vi "FES_CL_run.vi"() -> ()   [LabVIEW 2019]
uses:
  <vilib>/myRIO/Instrument Drivers/Onboard IO/DIO/typedefs/DIO Reference.ctl
  <vilib>/myRIO/Common/Instrument Driver Framework/Utilities/typedefs/myRIO Generic Hardware Reference.ctl
  <vilib>/myRIO/Common/Instrument Driver Framework/Utilities/typedefs/Hardware Version Enum.ctl
  <vilib>/myRIO/Common/Instrument Driver Framework/Utilities/typedefs/myRIO v1.0 Reference.ctl
  <vilib>/myRIO/Common/Instrument Driver Framework/Utilities/typedefs/Generic FPGA Reference.ctl
  <vilib>/myRIO/Common/Instrument Driver Framework/myRIO v1.0/DIO/typedefs/DIO Channels List.ctl
  <vilib>/myRIO/Common/Instrument Driver Framework/myRIO v1.0/DIO/typedefs/DIO Channels Enum.ctl
  <vilib>/userDefined/High Color/nirio_resource_hc.ctl
  <vilib>/Platform/TimedLoop/XDataNode/timing_clust.ctl
  <vilib>/Platform/TimedLoop/XDataNode/nitl_modes.ctl
  <vilib>/Platform/TimedLoop/XDataNode/wakeup.ctl
  <vilib>/myRIO/Instrument Drivers/Onboard IO/AI/typedefs/AI Reference.ctl
  <vilib>/myRIO/Common/Instrument Driver Framework/myRIO v1.0/AI/typedefs/AI Channels List.ctl
  <vilib>/myRIO/Common/Instrument Driver Framework/myRIO v1.0/AI/typedefs/AI Channels Enum.ctl
  <vilib>/myRIO/Common/Instrument Driver Framework/Utilities/typedefs/Analog Scaling Constants List.ctl
  <vilib>/myRIO/Common/Instrument Driver Framework/Utilities/typedefs/Analog Scaling Constants.ctl
  <vilib>/myRIO/Common/Instrument Driver Framework/Utilities/vis/Is FPGA Ref Available.vi
  <vilib>/myRIO/Common/Instrument Driver Framework/myRIO v1.0/DIO/vis/myRIO v1.1 Open DIO.vi
  <vilib>/myRIO/Instrument Drivers/Onboard IO/DIO/vis/Write.vi
  <vilib>/myRIO/Common/Instrument Driver Framework/myRIO v1.0/AI/vis/myRIO v1.1 Open AI.vi
  <vilib>/myRIO/Instrument Drivers/Onboard IO/AI/vis/Read.vi
  <vilib>/myRIO/Common/Instrument Driver Framework/Utilities/vis/Validate Channels.vi
  <vilib>/myRIO/Common/Instrument Driver Framework/myRIO v1.0/DIO/vis/myRIO v1.0 Reserve DIO.vi
  <vilib>/myRIO/Common/Instrument Driver Framework/myRIO v1.0/AI/vis/myRIO v1.0 Reserve AI.vi
  <vilib>/myRIO/Common/Instrument Driver Framework/myRIO v1.0/Resource Manager/vis/myRIO v1.0 Reserve Channel List.vi
  <vilib>/myRIO/Common/Instrument Driver Framework/myRIO v1.0/DIO/vis/myRIO v1.0 Build MUX Configuration DIO.vi
  <vilib>/myRIO/Common/Instrument Driver Framework/myRIO v1.0/AI/vis/myRIO v1.0 Build MUX Configuration AI.vi
  <vilib>/myRIO/Common/Instrument Driver Framework/myRIO v1.0/Resource Manager/vis/myRIO v1.0 Reserve Channel.vi
  <vilib>/myRIO/Common/Instrument Driver Framework/myRIO v1.0/Resource Manager/vis/myRIO v1.0 Unreserve Channel.vi
  <vilib>/myRIO/Common/Instrument Driver Framework/myRIO v1.0/Resource Manager/vis/myRIO v1.0 Create Configuration List.vi
  <vilib>/myRIO/Common/Instrument Driver Framework/myRIO v1.0/Resource Manager/vis/myRIO v1.0 Build Mutex Name.vi
  <vilib>/Utility/VariantDataType/GetNumericInfo.vi
  <vilib>/Utility/error.llb/Error Cluster From Error Code.vi
  <vilib>/myRIO/Common/Instrument Driver Framework/myRIO v1.0/myRIO v1.1 Open.vi
  <vilib>/myRIO/Common/Instrument Driver Framework/Utilities/vis/IO Manager.vi
  <vilib>/myRIO/Common/Instrument Driver Framework/Utilities/vis/Configuration Manager.vi
  <vilib>/myRIO/Common/Instrument Driver Framework/myRIO v1.0/Resource Manager/vis/myRIO v1.0 Configure IO.vi
  <vilib>/myRIO/Common/Instrument Driver Framework/myRIO v1.0/myRIO v1.0 Close.vi
  <vilib>/myRIO/Common/Instrument Driver Framework/myRIO v1.0/DIO/vis/myRIO v1.0 Write DIO.vi
  <vilib>/Utility/file.llb/Read Delimited Spreadsheet (DBL).vi
  FOS_CL/Global_vars.vi
  <vilib>/Utility/file.llb/Write Delimited Spreadsheet (DBL).vi
  <vilib>/myRIO/Common/Instrument Driver Framework/myRIO v1.0/AI/vis/myRIO v1.0 Get Scaling Constants AI.vi
  <vilib>/myRIO/Common/Instrument Driver Framework/myRIO v1.0/AI/vis/myRIO v1.0 Read AI.vi
  <vilib>/addons/control/pid/pid.llb/PID (DBL).vi
  <vilib>/myRIO/Express VI/Onboard IO/DO/DO Express VI.xnode
  <vilib>/myRIO/Instrument Drivers/Onboard IO/DIO/vis/myRIO DIO Open.xnode
  <vilib>/Platform/TimedLoop/XDataNode/XDataNode.xnode
  <vilib>/myRIO/Express VI/Onboard IO/AI/AI Express VI.xnode
  <vilib>/myRIO/Instrument Drivers/Onboard IO/AI/vis/myRIO AI Open.xnode
  <vilib>/myRIO/Instrument Drivers/Onboard IO/DIO/DIO.lvlib
  <vilib>/Platform/TimedLoop/XDataNode/XDNodeRunTimeDep.lvlib
  <vilib>/myRIO/Instrument Drivers/Onboard IO/AI/AI.lvlib
  <vilib>/ptbypt/NI_PtbyPt.lvlib
  <vilib>/addons/control/pid/NI_PID_pid.lvlib
panel:
  in  "Setup":T1(tab)
  in  "Sin Sq":bool
  in  "Ref freq (Hz)":dbl
  in  "Ref amp (mN)":dbl
  in  "Offset (mN)":dbl
  in  "output range":cluster{"output high":dbl, "output low":dbl}={"output high"=100.0, "output low"=-100.0} {"output low" format="%.2f"; "output high" format="%.2f"}
  in  "PID gains":T2={"proportional gain (Kc)"=1.0, "integral time (Ti, min)"=0.01, "derivative time (Td, min)"=0.0} {"derivative time (Td, min)" format="%.3f"; "integral time (Ti, min)" format="%.3f"; "proportional gain (Kc)" format="%.3f"}
  in  "Gyk":dbl
  in  "maxCS":dbl
  in  "minCS":dbl
  in  "Gff":dbl
  in  "y2":dbl
  in  "y1":dbl
  in  "x0":dbl
  in  "x1":dbl
  in  "x2":dbl
  in  "Offset2 (mN)":dbl
  in  "delta force (mN)":dbl
  in  "PW test (0-100%)":dbl
  in  "Stim Frequency (Hz)":dbl=39.0
  out "feedforward missed":dbl
  out "controller missed":dbl
  out "stim missed":dbl
  out "force reading missed":dbl
  out "save missed":dbl
  out "ref missed":dbl
  out "Fref":dbl[](graph)
  in  "File path":path=path "C:/Opto/fatigue_plantar2.txt"
  out "Control performance":cluster{"F ref":dbl, "raw F":dbl}(graph)
  out "Control signal":dbl(graph)
  out "forceInd":dbl
  out "Control signals":T3(graph)
  out "yk":dbl(graph)
  in  "Mode test CL":bool
  in  "stop":bool
  in  "Model off on":bool
  out "rawF":dbl[](graph)
  in  "stop test":bool
  out "controlSignal":dbl[](graph)
  out "controlVariable":dbl[](graph)
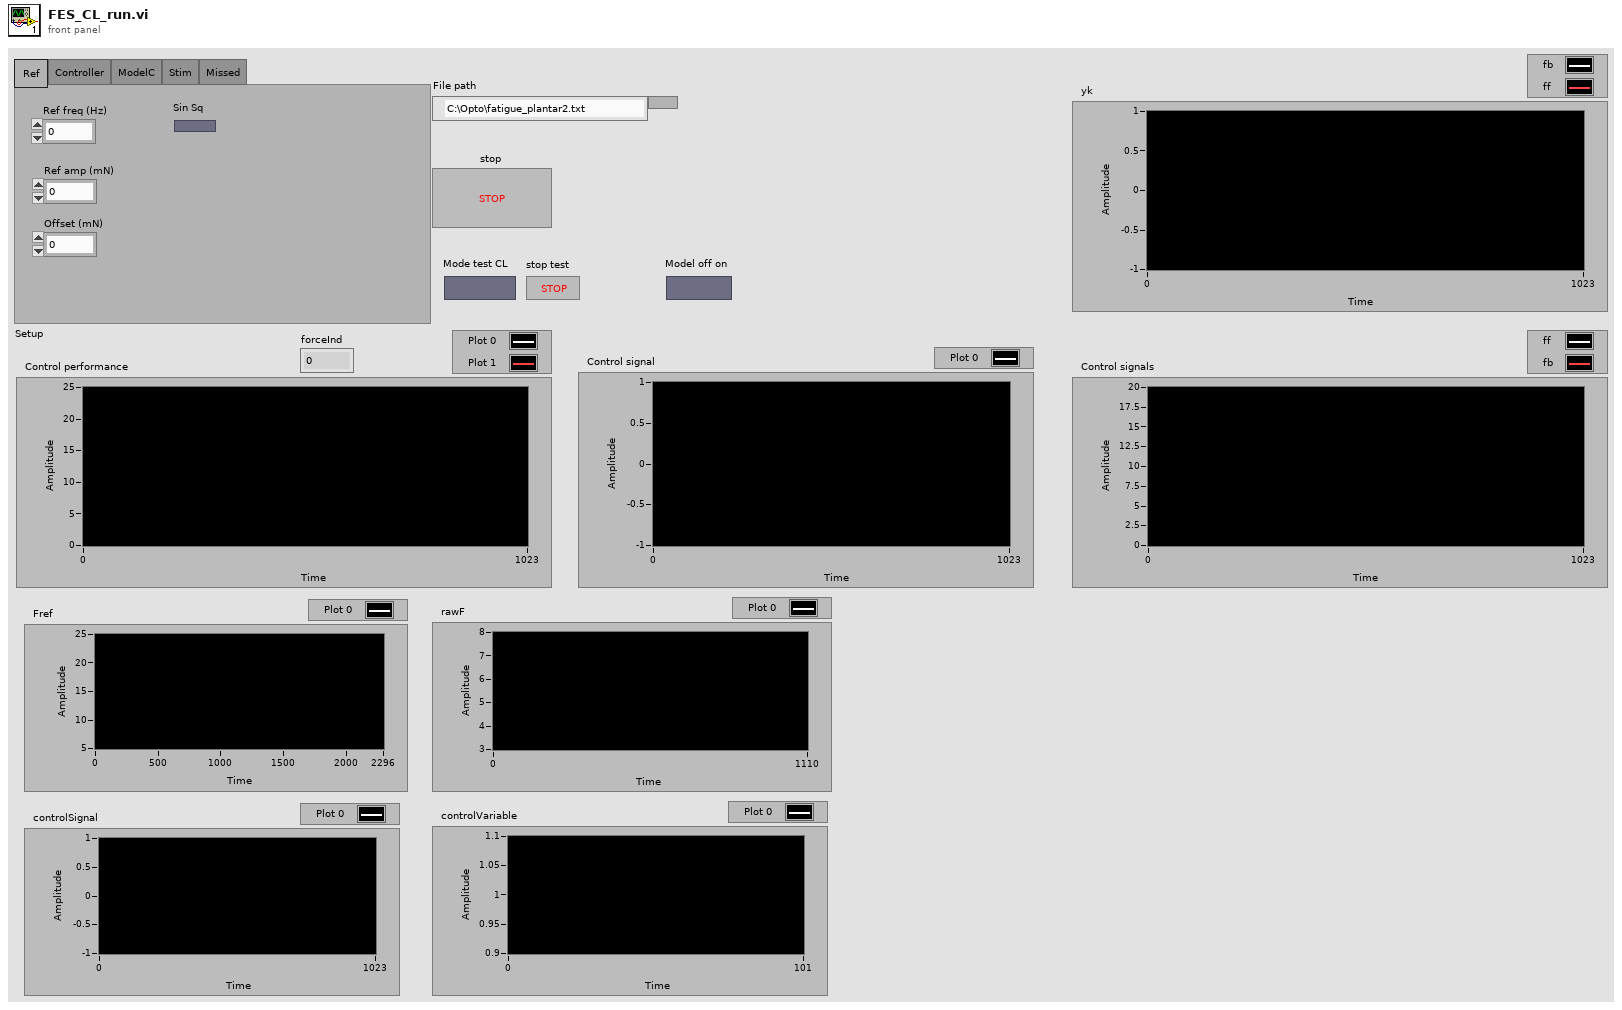
[diagram p1: front panel]
types:
  T1 = enum32{"Ref ", "Controller", "ModelC", "Stim", "Missed"}
  T2 = cluster{"proportional gain (Kc)":dbl, "integral time (Ti, min)":dbl, "derivative time (Td, min)":dbl}
  T3 = cluster{"control signal ff":dbl, "control signal fb":dbl}
  T4 = typedef "DIO.lvlib/DIO Reference.ctl" = cluster{"myRIO Reference":T5, "DIO Channels List":T9}
  T5 = typedef "myRIO Generic Hardware Reference.ctl" = cluster{"myRIO Model":T6, "myRIO Hardware Reference":T7}
  T6 = typedef "Hardware Version Enum.ctl" = enum16{"Unknown", "myRIO-1900", "myRIO-1950", "roboRIO", "NI ELVIS RIO CM", "ELVIS III"}
  T7 = typedef "myRIO v1.0 Reference.ctl" = cluster{"Generic FPGA Reference":T8, "Allow multiple opens":bool}
  T8 = typedef "Generic FPGA Reference.ctl" = refnum<k20>
  T9 = typedef "DIO Channels List.ctl" = T10[]
  T10 = typedef "DIO Channels Enum.ctl" = enum16{"Not Connected", "C/DIO0", "C/DIO1", "C/DIO2", "C/DIO3", "C/DIO4", "C/DIO5", "C/DIO6", "C/DIO7", "A/DIO0", "A/DIO1", "A/DIO2", "A/DIO3", "A/DIO4", "A/DIO5", "A/DIO6", "A/DIO7", "A/DIO8", "A/DIO9", "A/DIO10", "A/DIO11", "A/DIO12", "A/DIO13", "A/DIO14", "A/DIO15", "A/DIO16", "A/DIO17", "A/DIO18", "A/DIO19", "B/DIO0", "B/DIO1", "B/DIO2", "B/DIO3", "B/DIO4", "B/DIO5", "B/DIO6", "B/DIO7", "B/DIO8", "B/DIO9", "B/DIO10", "B/DIO11", "B/DIO12", "B/DIO13", "B/DIO14", "B/DIO15", "B/DIO16", "B/DIO17", "B/DIO18", "B/DIO19", "LED0", "LED1", "LED2", "LED3", "Button0", "DIO/DIO0", "DIO/DIO1", "DIO/DIO2", "DIO/DIO3", "DIO/DIO4", "DIO/DIO5", "DIO/DIO6", "DIO/DIO7", "DIO/DIO8", "DIO/DIO9", "SPI/CS0", "SPI/CS1", "SPI/CS2", "SPI/CS3", "LED RADIO (Green)", "LED RADIO (Red)", "LED COMM (Green)", "LED COMM (Red)", "LED MODE (Green)", "LED MODE (Red)"}
  T11 = typedef "nirio_resource_hc.ctl" = tag
  T12 = typedef "XDNodeRunTimeDep.lvlib/timing_clust.ctl" = cluster{"Expected End [f-1]":u64, "Actual End [f-1]":u64, "Finished Late? [f-1]":bool, "Expected End [i-1]":u64, "Actual End [i-1]":u64, "Finished Late? [i-1]":bool, "Expected Start [i]":u64, "Actual Start [i]":u64, "Expected Start [f]":u64, "Actual Start [f]":u64, "Source Name":string, "Structure Name":string, "Period":i64, "Deadline":i64, "Offset":i64, "Start":i64, "Priority":i32, "Timeout":i32, "Mode":T13, "Wakeup Reason":T14, "Error":errorcluster, "Source Type":string, "Secondary Source Type":string, "Global End Time":u64, "Global Start Time":u64, "Frame Duration":u64, "Iteration Duration":u64, "Assigned CPU":i32, "I/O Scan Engine Mode":u32}
  T13 = typedef "XDNodeRunTimeDep.lvlib/nitl_modes.ctl" = enum32{"No Change", "Process missed periods, maintain original phase", "Discard missed periods, maintain original phase", "Process missed periods, ignore original phase", "Discard missed periods, ignore original phase"}
  T14 = typedef "XDNodeRunTimeDep.lvlib/wakeup.ctl" = enum32{"Normal", "Aborted", "Asynchronous wakeup", "Timing source error", "Timed loop error", "Timeout"}
  T15 = typedef "AI.lvlib/AI Reference.ctl" = cluster{"myRIO Reference":T5, "AI Channels List":T16, "AI Scaling Constants List":T18}
  T16 = typedef "AI Channels List.ctl" = T17[]
  T17 = typedef "AI Channels Enum.ctl" = enum16{"Not Connected", "AudioIn/Left", "AudioIn/Right", "C/AI0", "C/AI1", "A/AI0", "A/AI1", "A/AI2", "A/AI3", "A/AI4", "A/AI5", "A/AI6", "A/AI7", "B/AI0", "B/AI1", "B/AI2", "B/AI3", "B/AI4", "B/AI5", "B/AI6", "B/AI7", "AI/AI0", "AI/AI1", "AI/AI2", "AI/AI3", "A/AI0 (DIFF)", "A/AI1 (DIFF)", "A/AI2 (DIFF)", "A/AI3 (DIFF)", "B/AI0 (DIFF)", "B/AI1 (DIFF)", "B/AI2 (DIFF)", "B/AI3 (DIFF)"}
  T18 = typedef "Analog Scaling Constants List.ctl" = T19[]
  T19 = typedef "Analog Scaling Constants.ctl" = cluster{"LSB Weight (Volts)":dbl, "Offset (Volts)":dbl, "Signed?":bool}
  T20 = cluster{"control signal fb":dbl, "control signal ff":dbl}
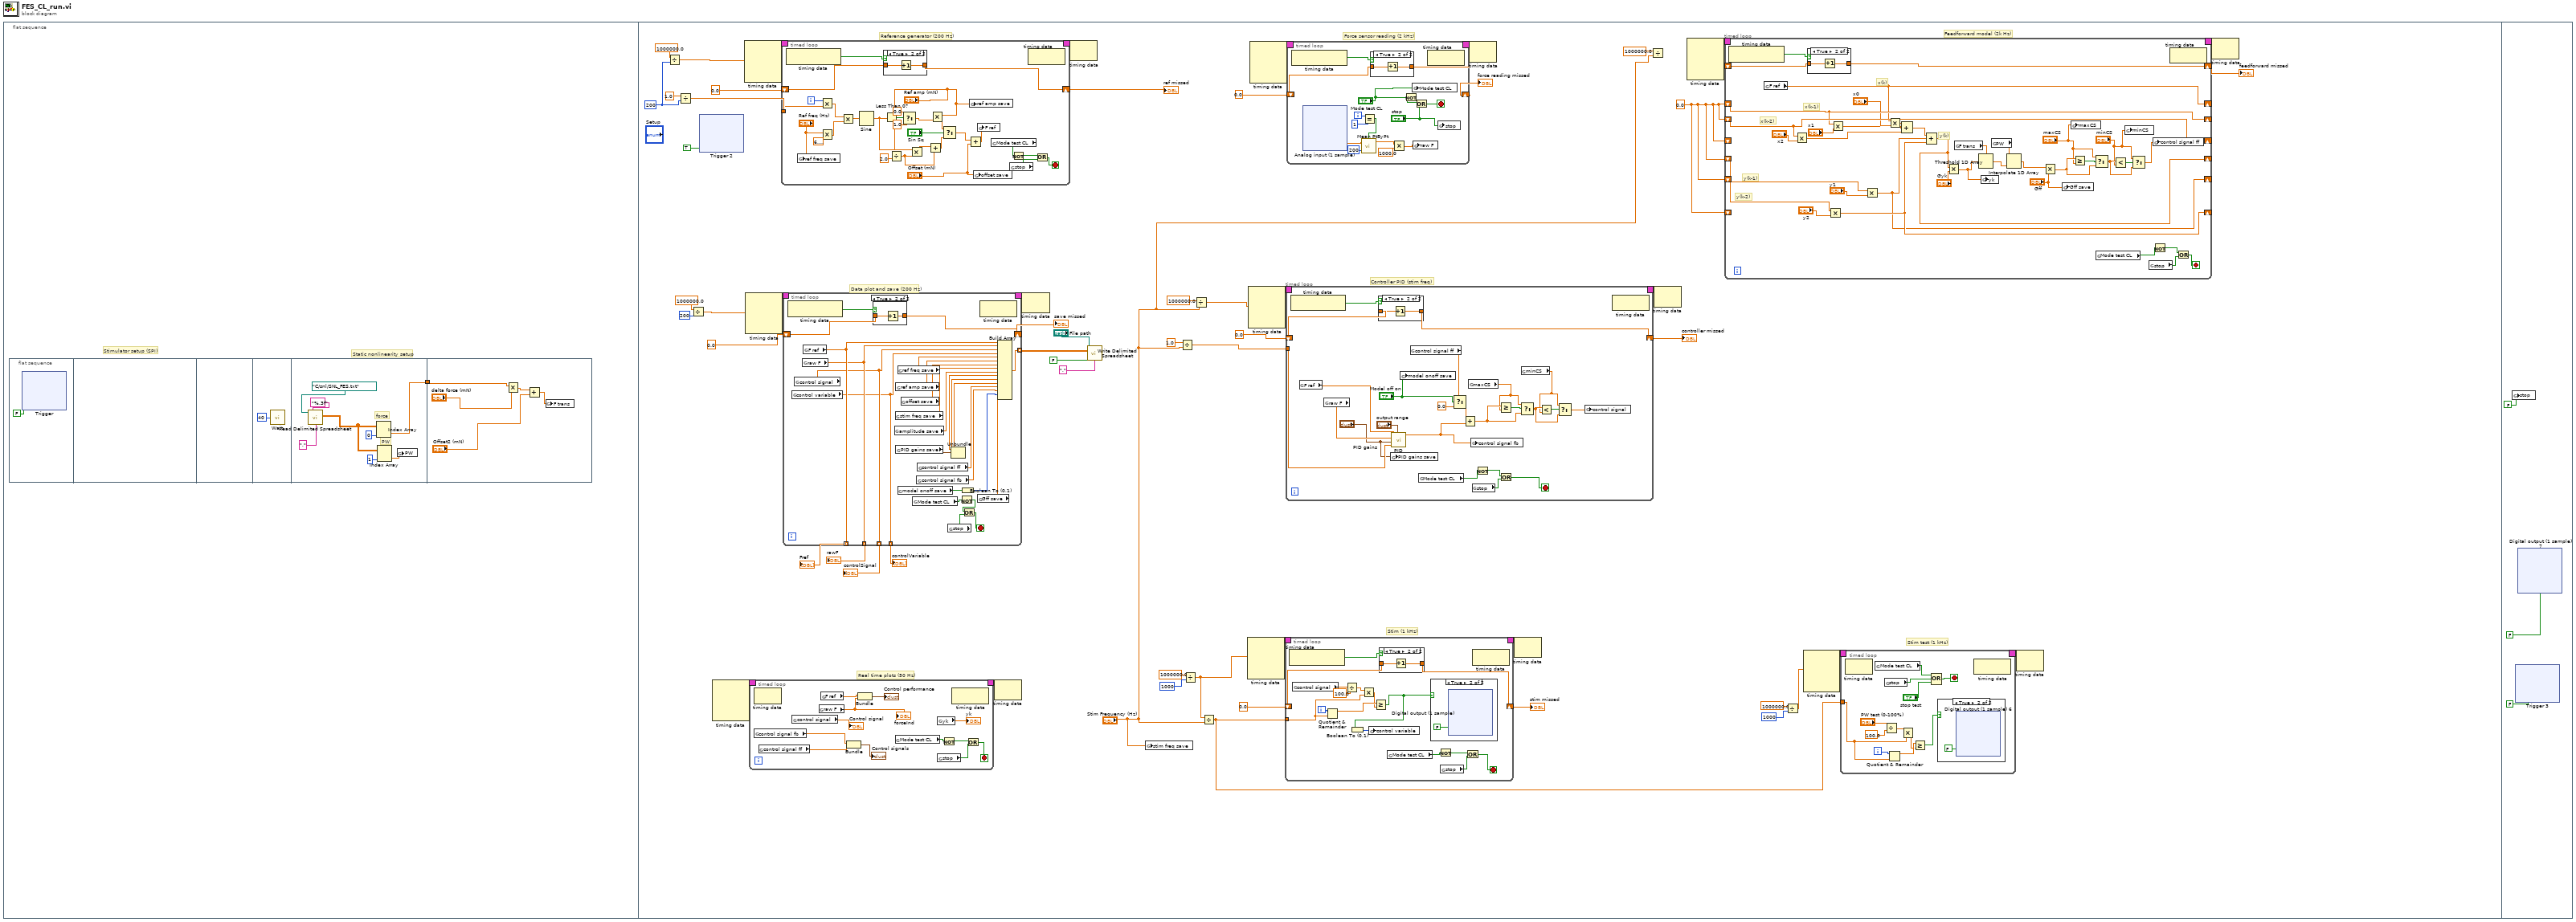
[diagram p0: block diagram]
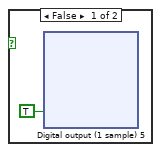
[diagram p3: hidden frame]
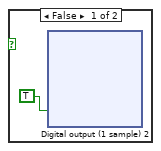
[diagram p5: hidden frame]
diagram:
  n1 = flat-sequence {
    frame #0 {
      # "Static nonlinearity setup"
      # "Stimulator setup (SPI)"
      n2 = flat-sequence {
        tunnel: [w39] -> w1
        tunnel: w1 -> [w50]
        frame #0 {
          n3 = xnode "Trigger"("C/DIO7 (DIO7)"=FALSE) -> ()  [unwired: 1 in, 1 out]
        }
        frame #1 {
        }
        frame #2 {
        }
        frame #3 {
          n4 = call "Wait"("Count(uSec)"=u32 40) -> ()  [unwired: 1 out]
        }
        frame #4 {
          # "PW"
          # "force"
          n5 = call-poly <vilib>:"Read Delimited Spreadsheet.vi"("file path (dialog if empty)"=path "C:/snl/SNL_FES.txt", "format (%.3f)"="%.3f", "delimiter (\\t)"="," ("delimiter (\\t)")) -> ("all rows"=w45:dbl[][])  [unwired: 7 in, 5 out]
          n6 = Index Array(array=w45, index (col)=0 ("disabled index (col)")) -> (element=w39:dbl[])  [unwired: 1 in]
          n7 = Index Array(array=w45, index (col)=1 ("disabled index (col)")) -> (element=w46:dbl[])  [unwired: 1 in]
          n8 = global write "Global_vars.vi" "PW"(w46) -> ()
        }
        frame #5 {
          n9 = Multiply(x=w50, y="delta force (mN)") -> (x*y=w51:dbl[])
          n10 = Add(x=w51, y="Offset2 (mN)") -> (x+y=w49:dbl[])
          n11 = global write "Global_vars.vi" "F trans"(w49) -> ()
        }
      }
    }
    frame #1 {
      w56 = 0.0 ("F ref")
      w101 = 200
      # "Feedforward model (2k Hz)"
      # "Stim test (1 kHz)"
      # "Stim (1 kHz)"
      # "Controller PID (stim freq)"
      # "Force sensor reading (2 kHz)"
      # "Real time plots (50 Hz)"
      # "Data plot and save (200 Hz)"
      # "Reference generator (200 Hz)"
      n12 = Divide(x=1000000.0, y=w101) -> (x/y=w103:dbl)
      n13 = Divide(x=1.0, y=w101) -> (x/y=w106:dbl)
      n14 = Divide(x=1000000.0, y=200) -> (x/y=w100:dbl)
      n15 = xnode "Trigger 2"("C/DIO7 (DIO7)"=TRUE) -> ()  [unwired: 1 in, 1 out]
      n16 = node-c288() -> (w93:T12)  [unwired: 4 in]
      n17 = node-c288(w103) -> (w109:T12)  [unwired: 3 in]
      n18 = node-c288(w100) -> (w105:T12)  [unwired: 3 in]
      n19 = timed-loop {
        timing: w93 -> [_]
        timing-out: [_] -> w92
        stop <- w481 stop-if-true
        n20 = node-c288() -> ()  [unwired: 1 in, 1 out]
        n21 = global read "Global_vars.vi" "control signal fb"() -> (w475:dbl)
        n22 = global read "Global_vars.vi" "control signal ff"() -> (w474:dbl)
        n23 = global read "Global_vars.vi" "control signal"() -> (→"Control signal":dbl)
        n24 = global read "Global_vars.vi" "raw F"() -> (w477:dbl)
        "forceInd" <- w477
        n25 = global read "Global_vars.vi" "F ref"() -> (w478:dbl)
        n26 = Bundle("control signal fb"=w475, "control signal ff"=w474) -> (→"Control signals":T20)  [unwired: 1 in]
        n27 = Bundle("F ref"=w478, "raw F"=w477) -> (→"Control performance":cluster{"F ref":dbl, "raw F":dbl})  [unwired: 1 in]
        n28 = global read "Global_vars.vi" "Mode test CL"() -> (w484:bool)
        n29 = global read "Global_vars.vi" "yk"() -> (→"yk":dbl)
        n30 = global read "Global_vars.vi" "stop"() -> (w482:bool)
        n31 = Not(x=w484) -> (.not. x?=w483:bool)
        n32 = node-c288() -> ()  [unwired: 1 in, 1 out]
        n33 = Or(x=w483, y=w482) -> (x .or. y?=w481:bool)
      }
      n34 = timed-loop {
        timing: w109 -> [_]
        timing-out: [_] -> w108
        tunnel: w106 -> [w551]
        shift-right: [w532] -> w90
        shift-left: 0.0 -> [w533]
        i -> [w552]
        stop <- w531 stop-if-true
        n35 = node-c288() -> (w534:bool)  [unwired: 1 in]
        n36 = global write "Global_vars.vi" "ref freq save"("Ref freq (Hz)") -> ()
        n37 = Multiply(x=w552, y=w551) -> (x*y=w550:dbl)
        n38 = Multiply(x="Ref freq (Hz)", y=6.283185307179586) -> (x*y=w549:dbl)
        n39 = Multiply(x=w550, y=w549) -> (x*y=w548:dbl)
        n40 = Sine(x=w548) -> (sin(x)=w539:dbl)
        n41 = case shown="True" w534 {
          tunnel: w533 -> [w554 w556]
          tunnel: [w554 w555] -> w532
          frame False {
          }
          frame True {
            n42 = Increment(x=w556) -> (x+1=w555:dbl)
          }
        }
        n43 = Less Than 0?(x=w539) -> (x < 0?=w547:bool)
        n44 = Divide(x="Ref amp (mN)", y=2.0) -> (x/y=w538:dbl)
        n45 = Select(t=0.0, s=w547, f=1.0) -> (s? t:f=w542:dbl)
        n46 = Multiply(x=w539, y=w538) -> (x*y=w537:dbl)
        n47 = Add(x=w537, y=w538) -> (x+y=w536:dbl)
        n48 = Multiply(x="Ref amp (mN)", y=w542) -> (x*y=w541:dbl)
        n49 = Select(t=w541, s="Sin Sq", f=w536) -> (s? t:f=w535:dbl)
        n50 = Add(x=w535, y="Offset (mN)") -> (x+y=w543:dbl)
        n51 = global write "Global_vars.vi" "ref amp save"("Ref amp (mN)") -> ()
        n52 = global write "Global_vars.vi" "offset save"("Offset (mN)") -> ()
        n53 = global write "Global_vars.vi" "F ref"(w543) -> ()
        n54 = global read "Global_vars.vi" "Mode test CL"() -> (w529:bool)
        n55 = global read "Global_vars.vi" "stop"() -> (w530:bool)
        n56 = Not(x=w529) -> (.not. x?=w528:bool)
        n57 = node-c288() -> ()  [unwired: 1 in, 1 out]
        n58 = Or(x=w528, y=w530) -> (x .or. y?=w531:bool)
      }
      "ref missed" <- w90
      n59 = timed-loop {
        timing: w105 -> [_]
        timing-out: [_] -> w104
        tunnel: [w511] -> w96 mode=indexing
        shift-right: [w512] -> w88
        shift-left: 0.0 -> [w513]
        tunnel: [w510] -> w69 mode=indexing
        tunnel: [w509] -> w68 mode=indexing
        tunnel: [w504] -> w61 mode=indexing
        tunnel: [w503] -> w60 mode=indexing
        stop <- w507 stop-if-true
        n60 = node-c288() -> (w514:bool)  [unwired: 1 in]
        n61 = global read "Global_vars.vi" "control variable"() -> (w503:dbl)
        n62 = global read "Global_vars.vi" "control signal"() -> (w504:dbl)
        n63 = global read "Global_vars.vi" "raw F"() -> (w510:dbl)
        n64 = global read "Global_vars.vi" "F ref"() -> (w511:dbl)
        n65 = case shown="True" w514 {
          tunnel: w513 -> [w515 w517]
          tunnel: [w515 w516] -> w512
          frame False {
          }
          frame True {
            n66 = Increment(x=w517) -> (x+1=w516:dbl)
          }
        }
        n67 = global read "Global_vars.vi" "amplitude save"() -> (w498:dbl)
        n68 = global read "Global_vars.vi" "stim freq save"() -> (w499:dbl)
        n69 = global read "Global_vars.vi" "ref amp save"() -> (w501:dbl)
        n70 = global read "Global_vars.vi" "PID gains save"() -> (w497:T2)
        n71 = global read "Global_vars.vi" "ref freq save"() -> (w502:dbl)
        n72 = global read "Global_vars.vi" "model onoff save"() -> (w491:bool)
        n73 = global read "Global_vars.vi" "offset save"() -> (w500:dbl)
        n74 = global read "Global_vars.vi" "Mode test CL"() -> (w505:bool)
        n75 = global read "Global_vars.vi" "control signal fb"() -> (w492:dbl)
        n76 = global read "Global_vars.vi" "control signal ff"() -> (w493:dbl)
        n77 = global read "Global_vars.vi" "stop"() -> (w508:bool)
        n78 = Unbundle(w497) -> ("proportional gain (Kc)"=w496:dbl, "integral time (Ti, min)"=w495:dbl, "derivative time (Td, min)"=w494:dbl)
        n79 = Not(x=w505) -> (.not. x?=w506:bool)
        n80 = Boolean To (0,1)(Boolean=w491) -> (0, 1=w490:i16)
        n81 = Or(x=w506, y=w508) -> (x .or. y?=w507:bool)
        n82 = global read "Global_vars.vi" "Gff save"() -> (w489:dbl)
        n83 = node-c288() -> ()  [unwired: 1 in, 1 out]
        n84 = Build Array(w511, w510, w504, w503, w502, w501, w500, w499, w498, w496, w495, w494, w493, w492, w490, w489) -> (w509:dbl[])
      }
      "Fref" <- w96
      "save missed" <- w88
      "rawF" <- w69
      "controlSignal" <- w61
      "controlVariable" <- w60
      n85 = node-c288(w92) -> ()  [unwired: 1 out]
      n86 = node-c288(w104) -> ()  [unwired: 1 out]
      n87 = node-c288(w108) -> ()  [unwired: 1 out]
      n88 = call-poly <vilib>:"Write Delimited Spreadsheet.vi"("file path (dialog if empty)"="File path", "2D data"=w68, "append to file? (new file:F)"=FALSE, "delimiter (\\t)"="," ("delimiter (\\t)")) -> ()  [unwired: 10 in, 2 out]
      n89 = global write "Global_vars.vi" "stim freq save"("Stim Frequency (Hz)") -> ()
      n90 = Divide(x=1.0, y="Stim Frequency (Hz)") -> (x/y=w72:dbl)
      n91 = Divide(x=1000000.0, y=1000) -> (x/y=w77:dbl)
      n92 = Divide(x=1000000.0, y="Stim Frequency (Hz)") -> (x/y=w52:dbl)
      n93 = Divide(x=w77, y="Stim Frequency (Hz)") -> (x/y=w62:dbl)
      n94 = node-c288(w77) -> (w81:T12)  [unwired: 3 in]
      n95 = node-c288(w52) -> (w83:T12)  [unwired: 3 in]
      n96 = node-c288() -> (w87:T12)  [unwired: 4 in]
      n97 = timed-loop {
        timing: w81 -> [_]
        timing-out: [_] -> w80
        tunnel: w62 -> [w293]
        shift-right: [w290] -> w75
        shift-left: 0.0 -> [w291]
        i -> [w292]
        stop <- w284 stop-if-true
        n98 = node-c288() -> (w289:bool)  [unwired: 1 in]
        n99 = global read "Global_vars.vi" "control signal"() -> (w296:dbl)
        n100 = Quotient & Remainder(x=w292, y=w293) -> (x-y*floor(x/y)=w282:dbl)  [unwired: 1 out]
        n101 = Divide(x=w296, y=100.0) -> (x/y=w294:dbl)
        n102 = Multiply(x=w294, y=w293) -> (x*y=w281:dbl)
        n103 = Greater Or Equal?(x=w282, y=w281) -> (x >= y?=w288:bool)
        n104 = Boolean To (0,1)(Boolean=w288) -> (0, 1=w287:i16)
        n105 = global write "Global_vars.vi" "control variable"(w287) -> ()
        n106 = case shown="True" w289 {
          tunnel: w291 -> [w297 w299]
          tunnel: [w297 w298] -> w290
          frame False {
          }
          frame True {
            n107 = Increment(x=w299) -> (x+1=w298:dbl)
          }
        }
        n108 = global read "Global_vars.vi" "Mode test CL"() -> (w283:bool)
        n109 = case shown="True" w288 {
          frame False {
            n110 = xnode "Digital output (1 sample) 2"("CH1 (C/DIO7 (DIO7))"=TRUE ("CH1 (A/DIO8 (Pin 27))")) -> ()  [unwired: 1 in, 1 out]
          }
          frame True {
            n111 = xnode "Digital output (1 sample)"("CH1 (C/DIO7 (DIO7))"=FALSE ("CH1 (A/DIO8 (Pin 27))")) -> ()  [unwired: 1 in, 1 out]
          }
        }
        n112 = Not(x=w283) -> (.not. x?=w285:bool)
        n113 = global read "Global_vars.vi" "stop"() -> (w286:bool)
        n114 = Or(x=w285, y=w286) -> (x .or. y?=w284:bool)
        n115 = node-c288() -> ()  [unwired: 1 in, 1 out]
      }
      "stim missed" <- w75
      n116 = timed-loop {
        timing: w83 -> [_]
        timing-out: [_] -> w82
        tunnel: w72 -> [w400]
        shift-right: [w397] -> w70
        shift-left: 0.0 -> [w398]
        stop <- w394 stop-if-true
        n117 = node-c288() -> (w399:bool)  [unwired: 1 in]
        n118 = global read "Global_vars.vi" "F ref"() -> (w389:dbl)
        n119 = global read "Global_vars.vi" "raw F"() -> (w401:dbl)
        n120 = case shown="True" w399 {
          tunnel: w398 -> [w403 w405]
          tunnel: [w403 w404] -> w397
          frame False {
          }
          frame True {
            n121 = Increment(x=w405) -> (x+1=w404:dbl)
          }
        }
        n122 = global write "Global_vars.vi" "PID gains save"("PID gains") -> ()
        n123 = call-poly <vilib>:"PID.vi"("output range"="output range", "dt (s)"=w400, "PID gains"="PID gains", "process variable"=w401, "setpoint"=w389) -> ("output"=w379:dbl)  [unwired: 5 in, 1 out]
        n124 = global write "Global_vars.vi" "model onoff save"("Model off on") -> ()
        n125 = global read "Global_vars.vi" "control signal ff"() -> (w388:dbl)
        n126 = global read "Global_vars.vi" "Mode test CL"() -> (w393:bool)
        n127 = Select(t=w388, s="Model off on", f=0.0) -> (s? t:f=w390:dbl)
        n128 = Add(x=w390, y=w379) -> (x+y=w382:dbl)
        n129 = global read "Global_vars.vi" "maxCS"() -> (w381:dbl)
        n130 = global write "Global_vars.vi" "control signal fb"(w379) -> ()
        n131 = global read "Global_vars.vi" "stop"() -> (w396:bool)
        n132 = Not(x=w393) -> (.not. x?=w395:bool)
        n133 = Greater Or Equal?(x=w382, y=w381) -> (x >= y?=w386:bool)
        n134 = Or(x=w395, y=w396) -> (x .or. y?=w394:bool)
        n135 = Select(t=w381, s=w386, f=w382) -> (s? t:f=w384:dbl)
        n136 = global read "Global_vars.vi" "minCS"() -> (w380:dbl)
        n137 = Less?(x=w384, y=w380) -> (x < y?=w385:bool)
        n138 = Select(t=w380, s=w385, f=w384) -> (s? t:f=w383:dbl)
        n139 = global write "Global_vars.vi" "control signal"(w383) -> ()
        n140 = node-c288() -> ()  [unwired: 1 in, 1 out]
      }
      "controller missed" <- w70
      n141 = timed-loop {
        timing: w87 -> [_]
        timing-out: [_] -> w86
        shift-right: [w421] -> w84
        shift-left: 0.0 -> [w422]
        i -> [w426]
        stop <- w418 stop-if-true
        n142 = node-c288() -> (w423:bool)  [unwired: 1 in]
        n143 = xnode "Analog input (1 sample)"() -> ("C/AI0 (AI0)"=w413:dbl)  [unwired: 1 in, 1 out]
        n144 = Equal?(x=w426, y=1) -> (x = y?=w424:bool)
        n145 = call <vilib>:"Mean PtByPt.vi"("x"=w413, "sample length"=200, "initialize"=w424) -> ("mean"=w415:dbl)  [unwired: 1 in, 1 out]
        n146 = case shown="True" w423 {
          tunnel: w422 -> [w428 w430]
          tunnel: [w428 w429] -> w421
          frame False {
          }
          frame True {
            n147 = Increment(x=w430) -> (x+1=w429:dbl)
          }
        }
        n148 = Multiply(x=w415, y=1000.0) -> (x*y=w414:dbl)
        n149 = Not(x="Mode test CL") -> (.not. x?=w420:bool)
        n150 = global write "Global_vars.vi" "Mode test CL"("Mode test CL") -> ()
        n151 = global write "Global_vars.vi" "raw F"(w414) -> ()
        n152 = Or(x=w420, y="stop") -> (x .or. y?=w418:bool)
        n153 = node-c288() -> ()  [unwired: 1 in, 1 out]
        n154 = global write "Global_vars.vi" "stop"("stop") -> ()
      }
      "force reading missed" <- w84
      n155 = node-c288(w86) -> ()  [unwired: 1 out]
      n156 = node-c288(w80) -> ()  [unwired: 1 out]
      n157 = Divide(x=1000000.0, y="Stim Frequency (Hz)") -> ()  [unwired: 1 out]
      n158 = node-c288(w82) -> ()  [unwired: 1 out]
      n159 = node-c288() -> (w58:T12)  [unwired: 4 in]
      n160 = timed-loop {
        timing: w58 -> [_]
        timing-out: [_] -> w57
        shift-right: [w145] -> w55
        shift-left: _ -> [w146]
        shift-right: [w111] -> _
        shift-left: w56 -> [w124]
        shift-right: [w124] -> _
        shift-left: w56 -> [w126]
        shift-right: [w126] -> _
        shift-left: w56 -> [_]
        shift-right: [w112] -> _
        shift-left: w56 -> [w134]
        shift-right: [w135] -> _
        shift-left: w56 -> [w139]
        shift-right: [w136] -> _
        shift-left: w56 -> [_]
        stop <- w141 stop-if-true
        # "y(k)"
        # "y(k-2)"
        # "y(k-1)"
        # "x(k-2)"
        # "x(k)"
        # "x(k-1)"
        n161 = node-c288() -> (w147:bool)  [unwired: 1 in]
        n162 = global read "Global_vars.vi" "F ref"() -> (w111:dbl)
        n163 = Multiply(x=w126, y="x2") -> (x*y=w119:dbl)
        n164 = case shown="True" w147 {
          tunnel: w146 -> [w148 w150]
          tunnel: [w148 w149] -> w145
          frame False {
          }
          frame True {
            n165 = Increment(x=w150) -> (x+1=w149:dbl)
          }
        }
        n166 = Multiply(x=w139, y="y2") -> (x*y=w136:dbl)
        n167 = Multiply(x=w124, y="x1") -> (x*y=w120:dbl)
        n168 = Multiply(x=w134, y="y1") -> (x*y=w135:dbl)
        n169 = Multiply(x=w111, y="x0") -> (x*y=w140:dbl)
        n170 = Compound Arithmetic op=ADD(w140, w120, w119) -> (w133:dbl)
        n171 = Compound Arithmetic op=ADD(w133, w135, w136) -> (w112:dbl)
        n172 = Multiply(x=w112, y="Gyk") -> (x*y=w110:dbl)
        n173 = global read "Global_vars.vi" "F trans"() -> (w138:dbl[])
        n174 = Threshold 1D Array(2:w110, 3:w138) -> (0:w132:dbl)  [unwired: 1 in]
        n175 = global write "Global_vars.vi" "yk"(w110) -> ()
        n176 = global read "Global_vars.vi" "PW"() -> (w137:dbl[])
        n177 = Interpolate 1D Array(1:w132, 2:w137) -> (0:w118:dbl)
        n178 = Multiply(x=w118, y="Gff") -> (x*y=w117:dbl)
        n179 = global write "Global_vars.vi" "Gff save"("Gff") -> ()
        n180 = global write "Global_vars.vi" "maxCS"("maxCS") -> ()
        n181 = Greater Or Equal?(x=w117, y="maxCS") -> (x >= y?=w131:bool)
        n182 = Select(t="maxCS", s=w131, f=w117) -> (s? t:f=w129:dbl)
        n183 = global read "Global_vars.vi" "Mode test CL"() -> (w144:bool)
        n184 = Less?(x=w129, y="minCS") -> (x < y?=w130:bool)
        n185 = global write "Global_vars.vi" "minCS"("minCS") -> ()
        n186 = Select(t="minCS", s=w130, f=w129) -> (s? t:f=w128:dbl)
        n187 = global read "Global_vars.vi" "stop"() -> (w142:bool)
        n188 = Not(x=w144) -> (.not. x?=w143:bool)
        n189 = global write "Global_vars.vi" "control signal ff"(w128) -> ()
        n190 = node-c288() -> ()  [unwired: 1 in, 1 out]
        n191 = Or(x=w143, y=w142) -> (x .or. y?=w141:bool)
      }
      "feedforward missed" <- w55
      n192 = Divide(x=1000000.0, y=1000) -> (x/y=w63:dbl)
      n193 = node-c288(w63) -> (w67:T12)  [unwired: 3 in]
      n194 = timed-loop {
        timing: w67 -> [_]
        timing-out: [_] -> w66
        tunnel: w62 -> [w198]
        i -> [w199]
        stop <- w191 stop-if-true
        n195 = node-c288() -> ()  [unwired: 1 in, 1 out]
        n196 = global read "Global_vars.vi" "Mode test CL"() -> (w194:bool)
        n197 = Divide(x="PW test (0-100%)", y=100.0) -> (x/y=w200:dbl)
        n198 = global read "Global_vars.vi" "stop"() -> (w193:bool)
        n199 = Quotient & Remainder(x=w199, y=w198) -> (x-y*floor(x/y)=w196:dbl)  [unwired: 1 out]
        n200 = Multiply(x=w200, y=w198) -> (x*y=w195:dbl)
        n201 = Greater Or Equal?(x=w196, y=w195) -> (x >= y?=w197:bool)
        n202 = Compound Arithmetic op=OR(w194, w193, "stop test") -> (w191:bool)
        n203 = case shown="True" w197 {
          frame False {
            n204 = xnode "Digital output (1 sample) 5"("CH1 (A/DIO8 (Pin 27))"=TRUE) -> ()  [unwired: 1 in, 1 out]
          }
          frame True {
            n205 = xnode "Digital output (1 sample) 6"("CH1 (A/DIO8 (Pin 27))"=FALSE) -> ()  [unwired: 1 in, 1 out]
          }
        }
        n206 = node-c288() -> ()  [unwired: 1 in, 1 out]
      }
      n207 = node-c288(w66) -> ()  [unwired: 1 out]
      n208 = node-c288(w57) -> ()  [unwired: 1 out]
    }
    frame #2 {
      n209 = global write "Global_vars.vi" "stop"(FALSE ("stop")) -> ()
      n210 = xnode "Trigger 3"("C/DIO7 (DIO7)"=FALSE) -> ()  [unwired: 1 in, 1 out]
      n211 = xnode "Digital output (1 sample) 7"("CH1 (A/DIO8 (Pin 27))"=FALSE) -> ()  [unwired: 1 in, 1 out]
    }
  }
